vi "Open_Create File.vi"(8 "error in (no error)":errorcluster, 11 "ConfigFile in":refnum<class "ConfigFile.lvclass">) -> (0 "error out":errorcluster, 1 "Operation":T1, 2 "Path":path, 3 "ConfigFile out":refnum<class "ConfigFile.lvclass">)   [LabVIEW 2017, in "ImportExport.lvlib" / "ConfigFile.lvclass"]
uses:
  ConfigFile.lvclass
  Operation.ctl
  ConfigFile.lvclass/ConfigFile.ctl
  ImportExport.lvlib
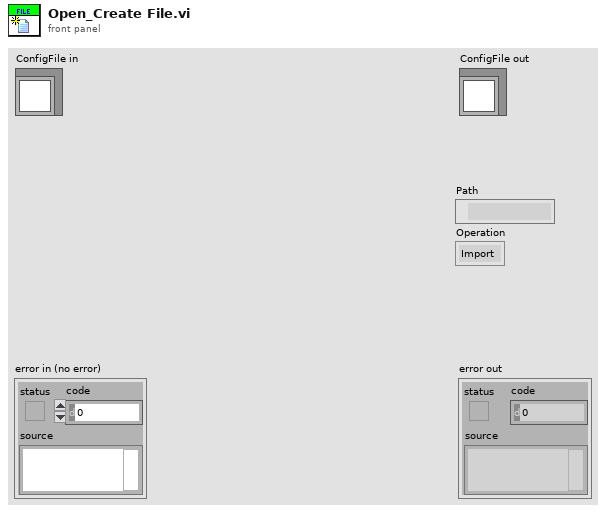
[diagram p1: front panel]
types:
  T1 = typedef "ImportExport.lvlib/Operation.ctl" = enum16{"Import", "Export"}
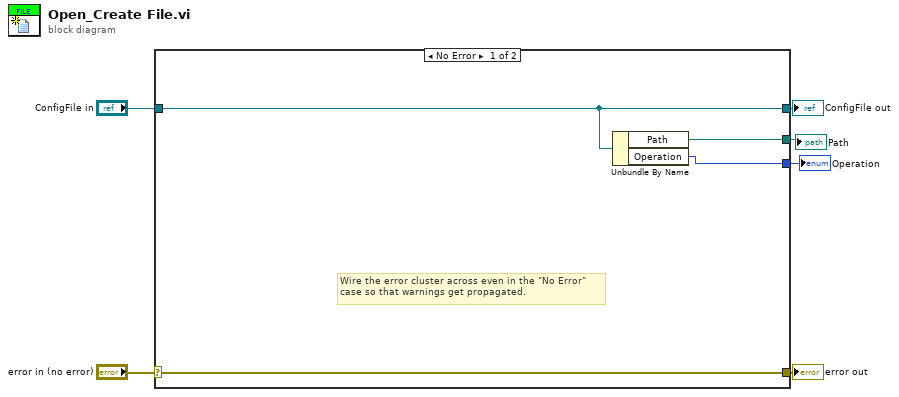
[diagram p0: block diagram]
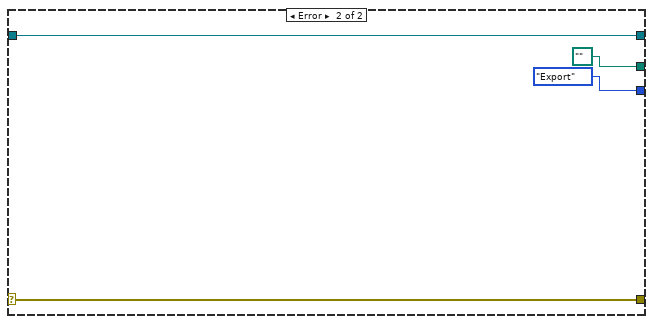
[diagram p2: hidden frame]
diagram:
  n1 = case shown="No Error" "error in (no error)" {
    selector: "error in (no error)" -> [w10 w14]
    tunnel: [w10 w14] -> w5
    tunnel: [w9 w13] -> w3
    tunnel: "ConfigFile in" -> [w9 w13]
    tunnel: [w8 path "" ("Path")] -> w2
    tunnel: [w7 Operation."Export" ("Operation")] -> w1
    frame No Error {
      # "Wire the error cluster across even in the \"No Error\"\ncase so that warnings get propagated."
      n2 = Unbundle By Name(w9) -> ("Path"=w8:path, "Operation"=w7:T1)
    }
    frame Error {
    }
  }
  "error out" <- w5
  "ConfigFile out" <- w3
  "Path" <- w2
  "Operation" <- w1
